vi "joystick+serial to robot.vi"() -> ()   [LabVIEW 2016]
uses:
  grSim/grSim Robot Command.ctl
  <vilib>/Instr/_visa.llb/VISA Configure Serial Port (Instr).vi
panel:
  out "Numeric 2":dbl
  out "String":string
  out "output cluster":T1
  out "return count":u32
  in  "stop":bool
  out "string":string
  out "error out":errorcluster
  in  "termination char\n(0xA = '\\n' = LF)":u8=10 format="%.0x"
  in  "VISA resource name":refnum<visa-resource-name>
  in  "Serial Settings":T2={"baud rate"=9600, "data bits"=8, "parity"=enum."None", "stop bits"=10, "flow control"=0} {"flow control" items=["None"=0, "XON/XOFF"=1, "RTS/CTS"=2, "DTR/DSR"=4]; "stop bits" items=["1.0"=10, "1.5"=15, "2.0"=20]; "data bits" min=5 max=8 step=1; "baud rate" items=["75"=75, "110"=110, "134"=134, "150"=150, "300"=300, "600"=600, "1200"=1200, "1800"=1800, "2400"=2400, "4800"=4800, "7200"=7200, "9600"=9600, "14400"=14400, "19200"=19200, "28800"=28800, "38400"=38400, "56000"=56000, "57600"=57600, "115200"=115200, "128000"=128000, "230400"=230400]}
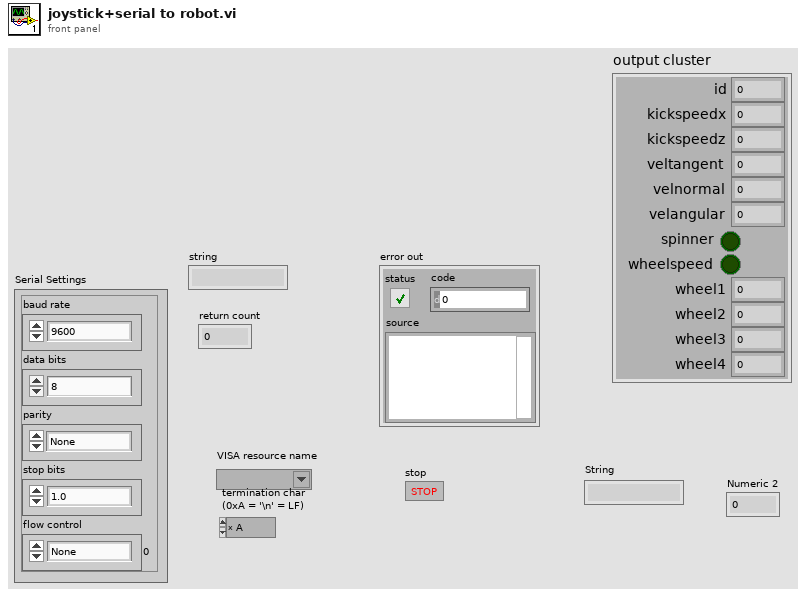
[diagram p1: front panel]
types:
  T1 = typedef "grSim Robot Command.ctl" = cluster{"id":u32, "kickspeedx":sgl, "kickspeedz":sgl, "veltangent":sgl, "velnormal":sgl, "velangular":sgl, "spinner":bool, "wheelspeed":bool, "wheel1":sgl, "wheel2":sgl, "wheel3":sgl, "wheel4":sgl}
  T2 = cluster{"baud rate":u32, "data bits":u16, "parity":enum16{"None", "Odd", "Even", "Mark", "Space"}, "stop bits":u16, "flow control":u16}
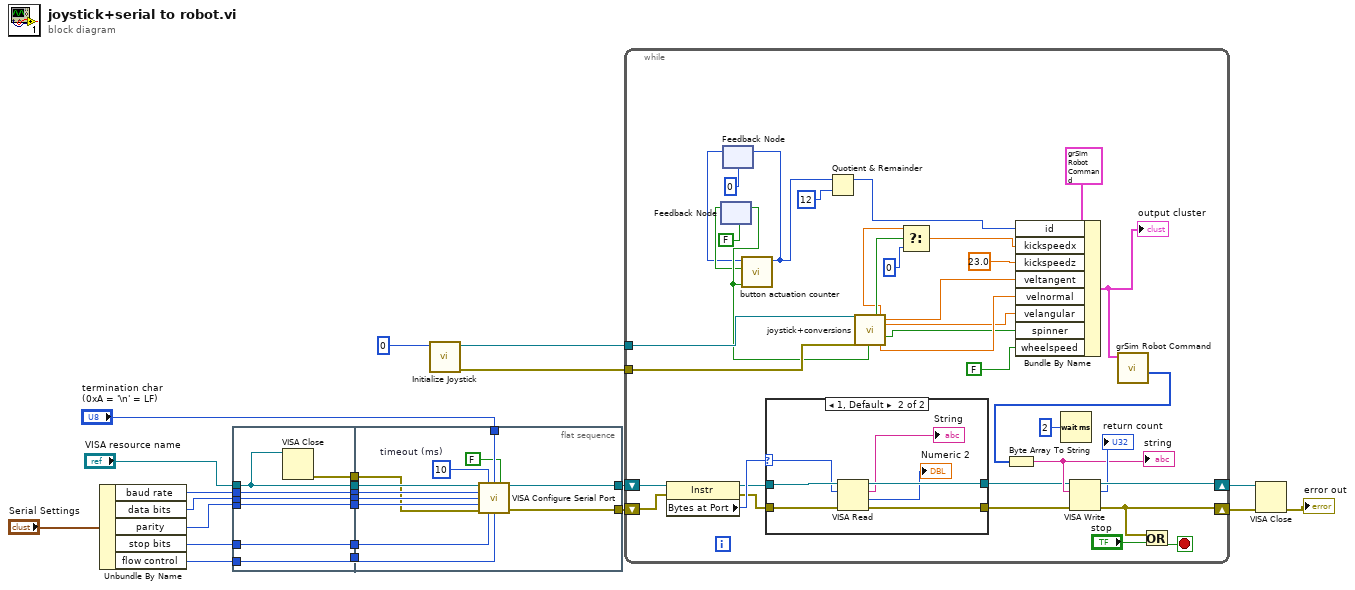
[diagram p0: block diagram]
diagram:
  n1 = Unbundle By Name("Serial Settings") -> ("baud rate"=w22:u32, "data bits"=w21:u16, "parity"=w20:enum16{"None", "Odd", "Even", "Mark", "Space"}, "stop bits"=w19:u16, "flow control"=w18:u16)
  n2 = flat-sequence {
    tunnel: "VISA resource name" -> [w25]
    tunnel: w18 -> [w26]
    tunnel: w19 -> [w27]
    tunnel: w20 -> [w28]
    tunnel: w21 -> [w29]
    tunnel: w22 -> [w30]
    tunnel: [w30] -> w7
    tunnel: [w29] -> w6
    tunnel: [w28] -> w5
    tunnel: [w27] -> w4
    tunnel: [w26] -> w3
    tunnel: [w25] -> w2
    tunnel: [w24] -> w1
    tunnel: "termination char\n(0xA = '\\n' = LF)" -> [w36]
    tunnel: [w34] -> w15
    tunnel: [w33] -> w13
    tunnel: w7 -> [w42]
    tunnel: w6 -> [w41]
    tunnel: w5 -> [w40]
    tunnel: w4 -> [w39]
    tunnel: w3 -> [w38]
    tunnel: w2 -> [w37]
    tunnel: w1 -> [w31]
    frame #0 {
      n3 = VISA Close(VISA resource name=w25) -> (error out=w24:errorcluster)  [unwired: 1 in]
    }
    frame #1 {
      w32 = u32 10  # timeout (ms)
      n4 = call-poly "VISA Configure Serial Port"("VISA resource name"=w37, "timeout (10sec)"=w32, "termination char\n(0xA = '\\n' = LF)"=w36, "Enable Termination\nChar (T)"=FALSE ("Enable Termination\nChar (T)"), "baud rate (9600)"=w42, "data bits (8)"=w41, "parity (0:none)"=w40, "error in (no error)"=w31, "stop bits (10: 1 bit)"=w39, "flow control (0:none)"=w38) -> ("VISA resource name out"=w34:refnum<visa-resource-name>, "error out"=w33:errorcluster)  [unwired: 4 in]
    }
  }
  n5 = call <vilib>:"Initialize Joystick.vi"("device index"=0) -> ("error out"=w8:errorcluster, "device ID"=w9:refnum<k1>)  [unwired: 9 in]
  n6 = while {
    shift-right: [w79] -> w14
    shift-left: w15 -> [w50]
    shift-right: [w75] -> w12
    shift-left: w13 -> [w49]
    tunnel: w9 -> [w65]
    tunnel: w8 -> [w64]
    stop <- w76 stop-if-true
    n7 = property class="Instr"(reference=w50, error in=w49) -> (reference out=w46:refnum<visa-resource-name>, error out=w47:errorcluster, "Bytes at Port"=w48:u32)
    n8 = feedback #1(FALSE) -> (w60:bool)
    n9 = feedback #2(0) -> (w58:i32)
    n10 = case shown="1, Default" w48 {
      selector: w48 -> [_ w82]
      tunnel: w47 -> [w80 w88]
      tunnel: [w80 w87] -> w52
      tunnel: w46 -> [w81 w86]
      tunnel: [w81 w85] -> w51
      frame 0 {
      }
      frame 1, Default {
        n11 = VISA Read(VISA resource name=w86, byte count=w82, error in (no error)=w88) -> (VISA resource name out=w85:refnum<visa-resource-name>, read buffer=→"String":string, return count=→"Numeric 2":u32, error out=w87:errorcluster)
      }
    }
    n12 = call "joystick+conversions.vi"("Refnum in"=w65, "error in (no error)"=w64) -> ("B pressed"=w61:bool, "v_radial"=w67:dbl, "A pressed"=w55:bool, "chute"=w53:dbl, "v_normal"=w69:dbl, "R*w"=w68:dbl, "Y pressed"=w45:bool)  [unwired: 9 in, 10 out]
    n13 = feedback-in #1(w61) -> ()
    n14 = call "button actuation counter.vi"("old count"=w58, "was button pressed ?"=w60, "button pressed now"=w61) -> ("new count"=w44:i32)  [unwired: 7 in]
    n15 = feedback-in #2(w44) -> ()
    n16 = Quotient & Remainder(x=w44, y=12) -> (x-y*floor(x/y)=w43:i32)  [unwired: 1 out]
    n17 = Select(t=w53, s=w55, f=0) -> (s? t:f=w54:dbl)
    n18 = Bundle By Name(cluster=T1 {"id"=0, "kickspeedx"=0.0, "kickspeedz"=0.0, "veltangent"=0.0, "velnormal"=0.0, "velangular"=0.0, "spinner"=FALSE, "wheelspeed"=FALSE, "wheel1"=0.0, "wheel2"=0.0, "wheel3"=0.0, "wheel4"=0.0} ("Robots"), "id"=w43, "kickspeedx"=w54, "kickspeedz"=sgl 23.0 ("kickspeedx"), "veltangent"=w67, "velnormal"=w69, "velangular"=w68, "spinner"=w45, "wheelspeed"=FALSE) -> (w63:T1)
    "output cluster" <- w63
    n19 = Wait (ms)(milliseconds to wait=u32 2) -> ()  [unwired: 1 out]
    n20 = call "grSim Robot Command.vi"("Robots"=w63) -> ("Array"=w72:u8[])  [unwired: 10 in]
    n21 = Byte Array To String(unsigned byte array=w72) -> (string=w73:string)
    "string" <- w73
    n22 = VISA Write(VISA resource name=w51, write buffer=w73, error in (no error)=w52) -> (VISA resource name out=w79:refnum<visa-resource-name>, return count=→"return count":u32, error out=w75:errorcluster)
    n23 = Or(x=w75, y="stop") -> (x .or. y?=w76:bool)
  }
  n24 = VISA Close(VISA resource name=w14, error in (no error)=w12) -> (error out=→"error out":errorcluster)
